vi "To String.vi"(8 "error in (no error)":errorcluster, 11 "OnTheFlyReport Config in":refnum<class "OnTheFlyReport Config.lvclass">) -> (0 "error out":errorcluster, 2 "data":string, 3 "OnTheFlyReport Config out":refnum<class "OnTheFlyReport Config.lvclass">)   [LabVIEW 2015, in "OnTheFlyReport Config.lvclass"]
uses:
  OnTheFlyReport Config.lvclass
  OnTheFlyReport Config.lvclass/OnTheFlyReport Config.ctl
  Report Formatters/Base Class/Config/Formatter Config.lvclass
  <vilib>/NI/Configuration Framework/serializable configuration/NISE_CEF_serializable configuration.lvclass
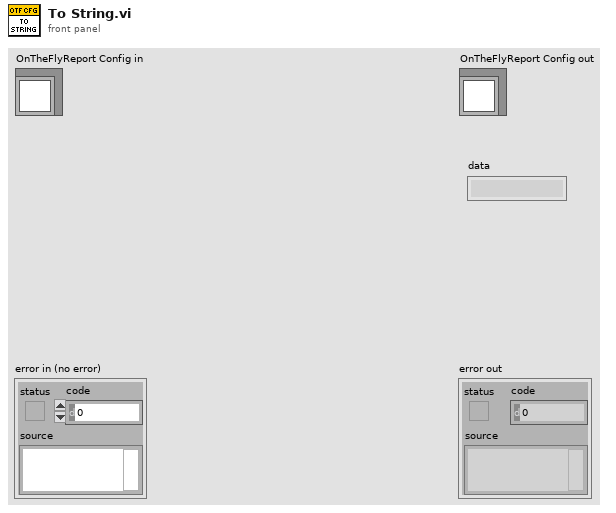
[diagram p1: front panel]
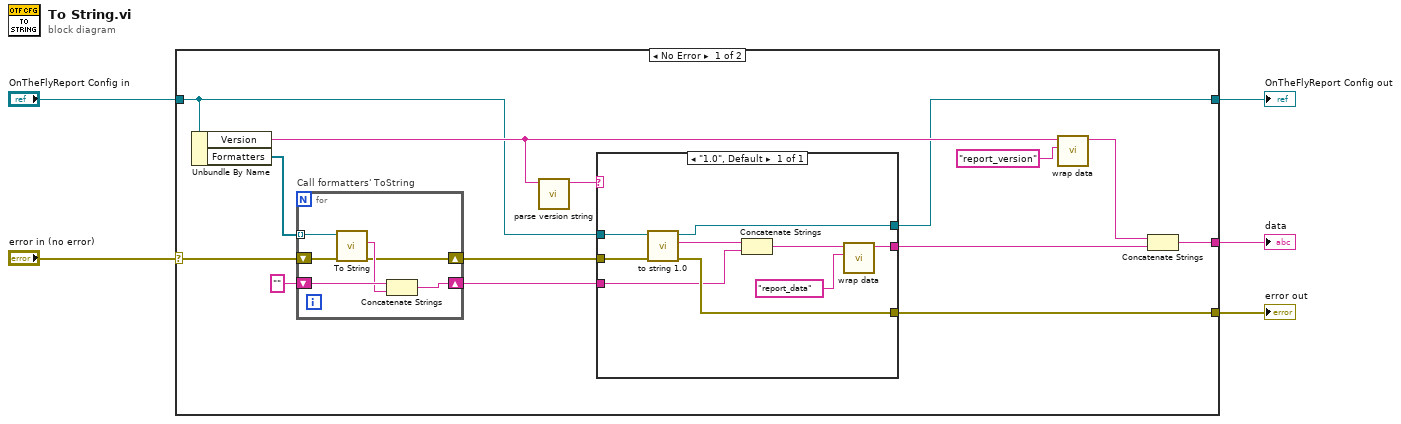
[diagram p0: block diagram]
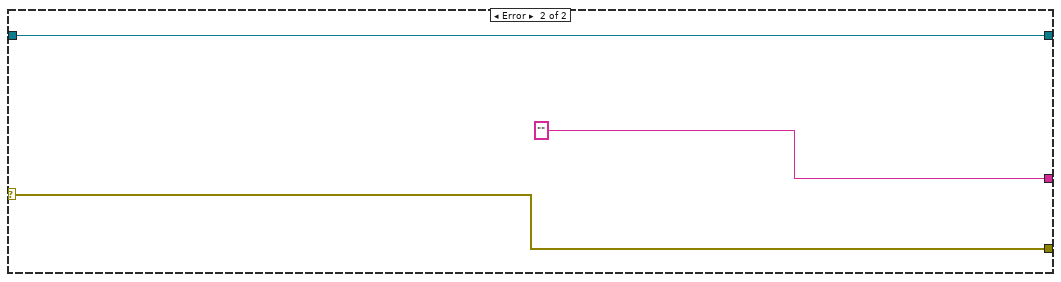
[diagram p2: hidden frame]
diagram:
  n1 = case shown="No Error" "error in (no error)" {
    selector: "error in (no error)" -> [w10 w37]
    tunnel: [w15 w37] -> w3
    tunnel: [w6 w36] -> w4
    tunnel: "OnTheFlyReport Config in" -> [w7 w36]
    tunnel: [w18 "" ("Version")] -> w1
    frame No Error {
      n2 = Unbundle By Name(w7) -> ("Version"=w14:string, "Formatters"=w9:refnum<class "Formatter Config.lvclass">[])
      n3 = for "Call formatters' ToString" {
        tunnel: w9 -> [w25] mode=indexing
        shift-right: [w20] -> w11
        shift-left: w10 -> [w24]
        shift-right: [w22] -> w8
        shift-left: "" ("data") -> [w23]
        n4 = call-dynamic "To String.vi"("error in (no error)"=w24, "Formatter Config in"=w25) -> ("error out"=w20:errorcluster, "data"=w21:string)  [unwired: 7 in, 1 out]
        n5 = Concatenate Strings(w23, w21) -> (w22:string)
      }
      n6 = call <vilib>:"parse version string.vi"("full version"=w14) -> ("major.minor version"=w13:string)  [unwired: 7 in, 3 out]
      n7 = case shown="\"1.0\", Default" w13 {
        tunnel: [w33] -> w16
        tunnel: [w32] -> w15
        tunnel: w8 -> [w30]
        tunnel: w11 -> [w29]
        tunnel: w7 -> [w27]
        tunnel: [w26] -> w6
        frame "1.0", Default {
          n8 = call-dynamic "to string 1.0.vi"("error in (no error)"=w29, "OnTheFlyReport Config in"=w27) -> ("error out"=w32:errorcluster, "wrapped data"=w28:string, "OnTheFlyReport Config out"=w26:refnum<class "OnTheFlyReport Config.lvclass">)  [unwired: 7 in]
          n9 = Concatenate Strings(w28, w30) -> (w31:string)
          n10 = call <vilib>:"wrap data.vi"("identifier"="report_data", "data to wrap"=w31) -> ("wrapped data"=w33:string)  [unwired: 9 in]
        }
      }
      n11 = call <vilib>:"wrap data.vi"("identifier"="report_version", "data to wrap"=w14) -> ("wrapped data"=w17:string)  [unwired: 9 in]
      n12 = Concatenate Strings(w17, w16) -> (w18:string)
    }
    frame Error {
    }
  }
  "error out" <- w3
  "OnTheFlyReport Config out" <- w4
  "data" <- w1
